vi "Creator Attributes.vi"(11 "TEMPLATE Actor in":refnum<class "TEMPLATE Actor.lvclass">) -> (2 "Creator Attributes":T1)   [LabVIEW 2020, in "_Template.lvlib" / "Templates.lvlib" / "TEMPLATE Actor.lvlib" / "TEMPLATE Actor.lvclass"]
uses:
  TEMPLATE Actor.lvclass
  jettl/jettl/Actor/Attributes.ctl
  jettl/jettl/Msg/Msg.lvclass
  jettl/jettl/Actor/Implemented Msgs.ctl
  TEMPLATE Actor.lvclass/TEMPLATE Actor.ctl
  jettl/jettl/Actor/Actor/Actor.lvclass
  jettl/jettl/Actor/Actor.lvlib
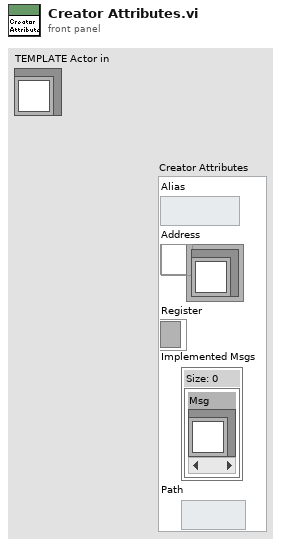
[diagram p1: front panel]
types:
  T1 = typedef "jettl.lvlib/Actor.lvlib/Attributes.ctl" = cluster{"Alias":string, "Address":refnum<user-event>, "Register":refnum<event-registration>, "Implemented Msgs":T2, "Path":path}
  T2 = typedef "jettl.lvlib/Actor.lvlib/Implemented Msgs.ctl" = set{refnum<class "Msg.lvclass">}
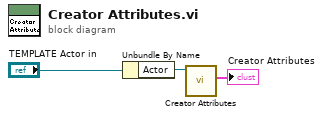
[diagram p0: block diagram]
diagram:
  n1 = Unbundle By Name("TEMPLATE Actor in") -> ("Actor"=w2:refnum<class "Actor.lvclass">)
  n2 = call-dynamic "Creator Attributes.vi"("Actor in"=w2) -> ("Creator Attributes"=→"Creator Attributes":T1)  [unwired: 10 in]
